vi "Actor Core.vi"(8 "error in":errorcluster, 11 "Test Actor in":refnum<class "Test Actor.lvclass">) -> (0 "error out":errorcluster, 3 "Actor out":refnum<class "Actor.lvclass">)   [LabVIEW 2017, in "Test Actor.lvclass"]
doc: "This actor will spawn new nested version of it's self if the levels to spawn is greater than zero.\n\nCopyright: MGI\nAuthored by: Derek Trepanier"
uses:
  Test Actor.lvclass
  C:/Program Files (x86)/National Instruments/LabVIEW 2017/vi.lib/ActorFramework/Actor/Actor.lvclass
  <vilib>/ActorFramework/Actor/Actor.lvclass
  <vilib>/ActorFramework/Actor/Actor.lvclass/Actor.ctl
  <vilib>/ActorFramework/Message Enqueuer/Message Enqueuer.lvclass/Message Enqueuer.ctl
  Test Actor.lvclass/Test Actor.ctl
  <vilib>/ActorFramework/Message Enqueuer/Init from Existing Queue.vi
  <vilib>/ActorFramework/Message Enqueuer/Message Enqueuer.lvclass
  Actor/Monitored Actor.lvclass
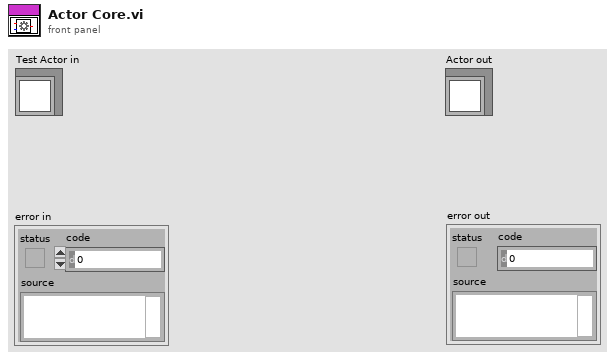
[diagram p1: front panel]
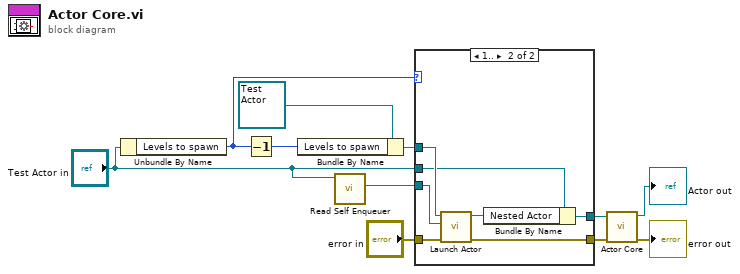
[diagram p0: block diagram]
diagram:
  n1 = Unbundle By Name("Test Actor in") -> ("Levels to spawn"=w5:i32)
  n2 = Decrement(x=w5) -> (x-1=w8:i32)
  n3 = Bundle By Name(cluster=refnum<class "Test Actor.lvclass"> refnum ("Test Actor in"), "Levels to spawn"=w8) -> (w7:refnum<class "Test Actor.lvclass">)
  n4 = call <vilib>:"Read Self Enqueuer.vi"("Actor"="Test Actor in") -> ("Self Enqueuer"=w6:refnum<class "Message Enqueuer.lvclass">)  [unwired: 10 in]
  n5 = case shown="1.." w5 {
    tunnel: w7 -> [_ w19]
    tunnel: w6 -> [_ w18]
    tunnel: [_ w17] -> w4
    tunnel: "error in" -> [_ w16]
    tunnel: "Test Actor in" -> [w12 w15]
    tunnel: [w12 w14] -> w1
    frame 0, Default {
    }
    frame 1.. {
      n6 = call <vilib>:"Launch Actor.vi"("error in (no error)"=w16, "Actor-to-Caller Enqueuer"=w18, "Actor"=w19) -> ("error out"=w17:errorcluster, "Caller-To-Actor Enqueuer"=w13:refnum<class "Message Enqueuer.lvclass">)  [unwired: 7 in]
      n7 = Bundle By Name(cluster=w15, "Nested Actor"=w13) -> (w14:refnum<class "Test Actor.lvclass">)
    }
  }
  n8 = call-parent "Actor Core.vi"("error in"=w4, "Actor in"=w1) -> ("error out"=→"error out":errorcluster, "Actor out"=→"Actor out":refnum<class "Actor.lvclass">)  [unwired: 8 in]
